vi "updateScreen.vi"(0 "reference":refnum<class "Graphics.lvclass">, 5 "error in (no error)":errorcluster) -> (14 "reference out":refnum<class "Graphics.lvclass">, 19 "error out":errorcluster)   [LabVIEW 2016, in "Graphics.lvclass"]
doc: "Updates the screen"
uses:
  <resource>/Framework/Providers/Open_GDS/UML/Graphics_class/Graphics.lvclass
panel:
  out "x-y":u32
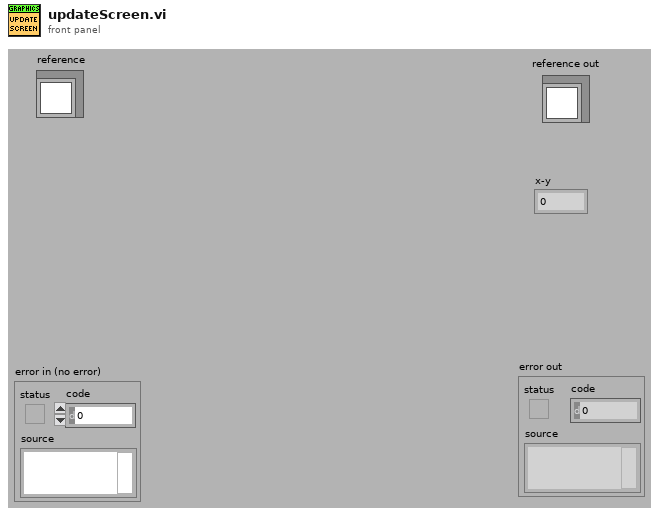
[diagram p1: front panel]
types:
  T1 = typedef "Graphics.lvclass/ObjectAttributes.ctl" = cluster{"drawColor":u32, "backgroundColor":u32, "font":T2, "fontType":T3, "picture":picture, "stroke":T4, "scaleX":dbl, "scaleY":dbl, "screenRef":refnum<vi>, "offsetX":dbl, "offsetY":dbl}
  T2 = typedef "Graphics.lvclass/FontType.ctl" = cluster{"Font Name:":string, "Size":i16, "Strikeout?":bool, "Italic?":bool, "Underline?":bool, "Outline?":bool, "Shadow?":bool, "Bold?":bool}
  T3 = typedef "Graphics.lvclass/LvFontType.ctl" = enum16{"User-specified Font", "Application Font", "System Font", "Dialog Font"}
  T4 = typedef "Graphics.lvclass/StrokeType.ctl" = enum16{"USE_DEFAULT", "SOLID", "DOTTED"}
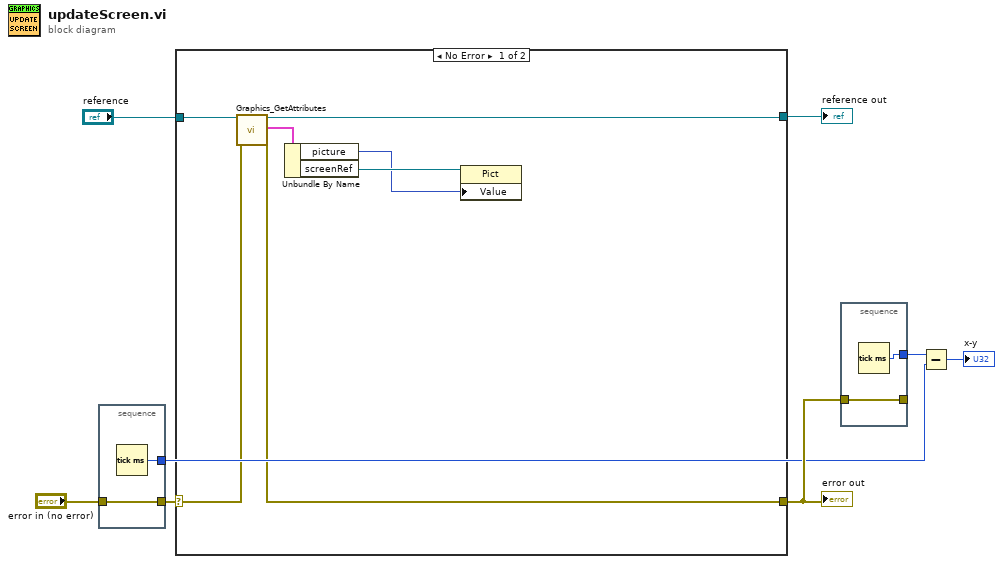
[diagram p0: block diagram]
diagram:
  n1 = stacked-sequence {
    tunnel: "error in (no error)" -> [w10]
    tunnel: [w10] -> w5
    tunnel: [w9] -> w2
    frame #0 {
      n2 = Tick Count (ms)() -> (millisecond timer value=w9:u32)
    }
  }
  n3 = case shown="No Error" w5 {
    selector: w5 -> [w17 w18]
    tunnel: "reference" -> [w16 w19]
    tunnel: [w14 w18] -> w4
    tunnel: [w15 w19] -> w7
    frame No Error {
      n4 = call <resource>:"Graphics_GetAttributes.vi"("reference in"=w16, "error in (no error)"=w17) -> ("reference out"=w15:refnum<class "Graphics.lvclass">, "Data"=w11:T1, "error out"=w14:errorcluster)  [unwired: 1 in, 14 out]
      n5 = Unbundle By Name(w11) -> ("picture"=w12:picture, "screenRef"=w13:refnum<vi>)
      n6 = property class="Pict"(reference=w13, "Value"=w12) -> ()  [unwired: 1 in, 2 out]
    }
    frame Error {
    }
  }
  "reference out" <- w7
  "error out" <- w4
  n7 = stacked-sequence {
    tunnel: w4 -> [w21]
    tunnel: [w21] -> _
    tunnel: [w20] -> w3
    frame #0 {
      n8 = Tick Count (ms)() -> (millisecond timer value=w20:u32)
    }
  }
  n9 = Subtract(x=w3, y=w2) -> (x-y=→"x-y":u32)
